vi "GetPoint.vi"(7 "Mode":enum16{"Read", "Configure"}(ring), 10 "Settings":T1={"Scan mode"=enum."Points", "NumPoints"=0, "NumReps"=0, "Motion Increment"=0, "NumMotionPoints"=0, "VolumeSettings"={"XStart"=0, "XEnd"=0, "XNum"=1, "YStart"=0, "YEnd"=0, "YNum"=1, "ZStart"=0, "ZEnd"=0, "ZNum"=1}} {"VolumeSettings"."ZNum" min=1 max=10000; "VolumeSettings"."YNum" min=1 max=10000; "VolumeSettings"."XNum" min=1 max=10000}, 11 "Sample Number":u32) -> (0 "RepNum":u32, 1 "Point Num":u32, 2 "Done":bool, 3 "Point":cluster{"X":i32, "Y":i32, "Z":i32}, 5 "Frame Start":bool)   [LabVIEW 2014]
uses:
  <vilib>/rvi/Emulation/niFpgaGetClockAttributes.vi
  <vilib>/rvi/Emulation/niFpgaSctlEmulationGetInTimedLoop.vi
  <vilib>/rvi/Emulation/niFpgaEmulationReportErrorSimple.vi
  <vilib>/rvi/Emulation/niFpgaCriticalErrorInLSC.vi
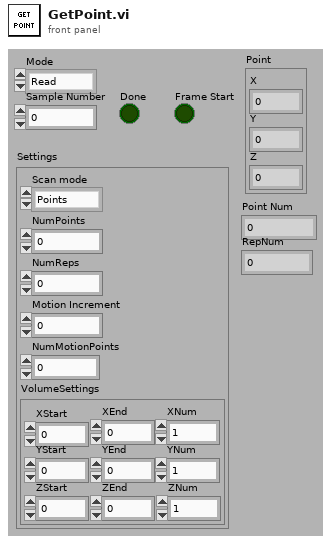
[diagram p1: front panel]
types:
  T1 = cluster{"Scan mode":enum16{"Points", "Volume", "Idle"}, "NumPoints":u32, "NumReps":u32, "Motion Increment":u32, "NumMotionPoints":u32, "VolumeSettings":cluster{"XStart":i32, "XEnd":i32, "XNum":i32, "YStart":i32, "YEnd":i32, "YNum":i32, "ZStart":i32, "ZEnd":i32, "ZNum":i32}}
  T2 = cluster{"XStart":i32, "XEnd":i32, "XNum":i32, "YStart":i32, "YEnd":i32, "YNum":i32, "ZStart":i32, "ZEnd":i32, "ZNum":i32}
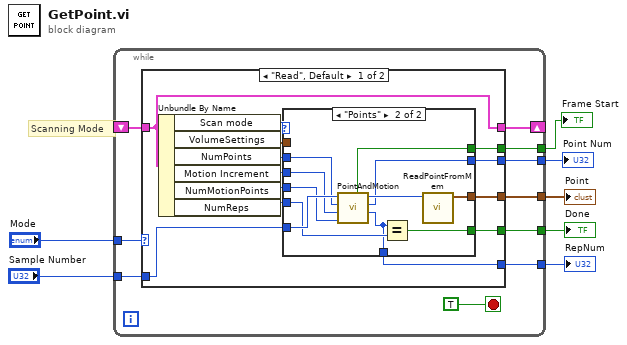
[diagram p0: block diagram]
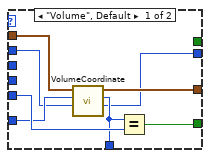
[diagram p2: hidden frame]
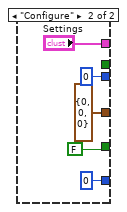
[diagram p3: hidden frame]
diagram:
  # "Scanning Mode"
  n1 = while {
    tunnel: "Mode" -> [w16]
    shift-right: [w15] -> _
    shift-left: _ -> [w14]
    tunnel: "Sample Number" -> [w13]
    tunnel: [w12] -> w5
    tunnel: [w11] -> w4
    tunnel: [w10] -> w3
    tunnel: [w9] -> w2
    tunnel: [w8] -> w1
    stop <- TRUE stop-if-true
    n2 = case shown="\"Read\", Default" w16 {
      tunnel: [w29 "Settings"] -> w15
      tunnel: w14 -> [w29 _]
      tunnel: w13 -> [w30 _]
      tunnel: [w23 cluster{"X":i32, "Y":i32, "Z":i32} {"X"=0, "Y"=0, "Z"=0} ("Point")] -> w12
      tunnel: [w21 FALSE] -> w11
      tunnel: [w20 u32 0 ("Point Num")] -> w10
      tunnel: [w19 u32 0 ("Rep Num")] -> w9
      tunnel: [w18 _] -> w8
      frame "Read", Default {
        n3 = Unbundle By Name(w29) -> ("Scan mode"=w28:enum16{"Points", "Volume", "Idle"}, "VolumeSettings"=w27:T2, "NumPoints"=w26:u32, "Motion Increment"=w25:u32, "NumMotionPoints"=w24:u32, "NumReps"=w22:u32)
        n4 = case shown="\"Points\"" w28 {
          tunnel: w30 -> [w34 w48]
          tunnel: [w38 w49] -> w23
          tunnel: w27 -> [w37 _]
          tunnel: w26 -> [w31 w47]
          tunnel: w25 -> [_ w46]
          tunnel: w24 -> [_ w45]
          tunnel: w22 -> [w36 w43]
          tunnel: [w35 w42] -> w21
          tunnel: [w32 w41] -> w20
          tunnel: [w33 w40] -> w19
          tunnel: [_ w39] -> w18
          frame "Volume", Default {
            n5 = call "VolumeCoordinate.vi"("NumPoints"=w31, "SampleNum"=w34, "Scan Settings"=w37) -> ("PointNum"=w32:u32, "RepNum"=w33:u32, "Point"=w38:cluster{"X":i32, "Y":i32, "Z":i32})  [unwired: 6 in]
            n6 = Equal?(x=w33, y=w36) -> (x = y?=w35:bool)
          }
          frame "Points" {
            n7 = call "PointAndMotion.vi"("Motion Points"=w45, "Motion Increment"=w46, "Num Points"=w47, "Sample Num"=w48) -> ("Rep Num"=w40:u32, "Point Num"=w41:u32, "Point Location"=w44:u32, "Frame Start"=w39:bool)  [unwired: 3 in, 1 out]
            n8 = Equal?(x=w40, y=w43) -> (x = y?=w42:bool)
            n9 = call "ReadPointFromMem.vi"("PointNum"=w44) -> ("Point"=w49:cluster{"X":i32, "Y":i32, "Z":i32})  [unwired: 10 in]
          }
        }
      }
      frame "Configure" {
      }
    }
  }
  "Point" <- w5
  "Done" <- w4
  "Point Num" <- w3
  "RepNum" <- w2
  "Frame Start" <- w1
